vi "get_listbox_items.vi"(11 "Volumes in":refnum<class "Volumes.lvclass">) -> (2 "listbox items":string[][](array[string]), 3 "Volumes out":refnum<class "Volumes.lvclass">)   [LabVIEW 2024, in "CLZ_to_ComicVine.lvlib" / "Volumes.lvclass"]
uses:
  Volumes.lvclass
  Volumes.lvclass/Volumes.ctl
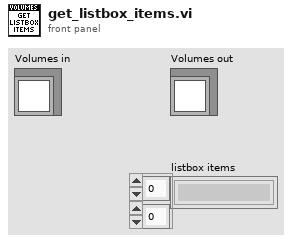
[diagram p1: front panel]
types:
  T1 = typedef "CLZ_to_ComicVine.lvlib/Volumes.lvclass/volume--cluster.ctl" = cluster{"id":i32, "name":string, "issue set":set{string}, "matched":bool}
  T2 = cluster{"name":string, "f":string, string, string}
  T3 = cluster{"name":string, "f":string, string, string}[]
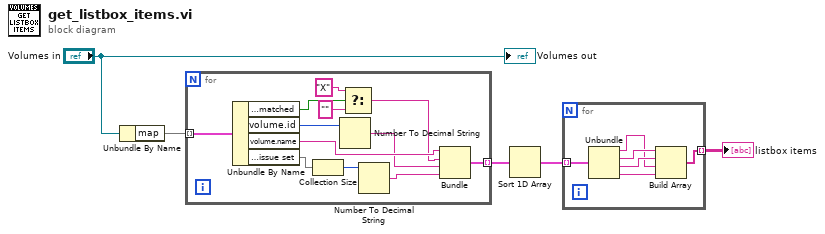
[diagram p0: block diagram]
diagram:
  n1 = Unbundle By Name("Volumes in") -> ("map"=w5:map{i32, T1})
  n2 = for {
    tunnel: w5 -> [w17] mode=indexing
    tunnel: [w6] -> w3 mode=indexing
    n3 = Unbundle By Name(w17) -> ("volume.matched"=w14:bool, "volume.id"=w13:i32, "volume.name"=w10:string, "volume.issue set"=w12:set{string})
    n4 = Collection Size(1:w12) -> (0:w11:i32)
    n5 = Number To Decimal String(number=w13) -> (decimal integer string=w8:string)  [unwired: 1 in]
    n6 = Select(t="X", s=w14, f="") -> (s? t:f=w9:string)
    n7 = Number To Decimal String(number=w11) -> (decimal integer string=w7:string)  [unwired: 1 in]
    n8 = Bundle("name"=w10, "f"=w9, w8, w7) -> (w6:T2)  [unwired: 1 in]
  }
  n9 = Sort 1D Array(array=w3) -> (sorted array=w2:T3)
  n10 = for {
    tunnel: w2 -> [w23] mode=indexing
    tunnel: [w18] -> w1 mode=indexing
    n11 = Unbundle(w23) -> ("name"=w19:string, "f"=w22:string, w21:string, w20:string)
    n12 = Build Array(w22, w21, w19, w20) -> (w18:string[])
  }
  "listbox items" <- w1
  "Volumes out" <- "Volumes in"
